vi "BonOMM-SAOMM.Test.vi"() -> ()   [LabVIEW 2011] (continued)
                n3732 = property on="ImgArray" class="IntGraph (strict)"("Cursor.Cursor Position"=w1831) -> ()  [unwired: 2 in, 2 out]
              }
              event "StartServo": Value Change {
                # "Permet l'annulation des\ncommandes de guidage."
                n3733 = event-data() -> ()  [unwired: 1 in, 5 out]
                n3734 = local write "StartServo"(FALSE ("StartServo")) -> ()
                n3735 = local write "GuidingCancel"(FALSE ("GuidingCancel")) -> ()
                n3736 = Less Or Equal?(x="Mode", y=u16 3) -> (x <= y?=w1870:bool)
                n3737 = case shown="True" w1870 {
                  tunnel: "Mode" -> [_ w1876]
                  frame False {
                    # "Ici, ce sera le mode \"calibration\" ..."
                  }
                  frame True {
                    # "Pour lancer le guidage traditionnel, il suffit de\nmettre l'indicateur d'activation à \"vrai\" ... on en\nprofite aussi pour remettre le compteur à zéro."
                    n3738 = flat-sequence {
                      tunnel: w1876 -> [w1879]
                      tunnel: [w1879] -> w1875
                      tunnel: [w1877] -> w1872
                      tunnel: w1875 -> [w1895]
                      tunnel: [w1895] -> w1874
                      tunnel: w1872 -> [w1894]
                      tunnel: w1874 -> [w1906]
                      tunnel: [w1906] -> w1873
                      tunnel: w1873 -> [w1944]
                      frame #0 {
                        w1882 = T17."Disabled and Grayed Out" ("Disabled")
                        w1884 = T17."Disabled" ("Disabled")
                        # "Si le mode est calibration\nC'est qu'on ajuste la collimation"
                        # "Lors de offset, un fichier sera créer à chaque fois :("
                        n3739 = local read "LoggingTimeStamp"() -> (→"GraphTimeStamp":dbl)
                        n3740 = Get Date/Time In Seconds() -> (seconds since 1Jan1904=w1888:timestamp)
                        n3741 = To Double Precision Float(number=w1888) -> (double precision float=w1889:dbl)
                        n3742 = call "GetPathFromTimeStamp.vi"("UTC Time"=TRUE, "LocalTimeStamp"=w1889, "Changement de date à midi ?"=TRUE) -> ("Time String"=w1886:string)  [unwired: 11 in, 1 out]
                        n3743 = Concatenate Strings(w1886, ".gud") -> (→"TrackLogFilename":string)
                        n3744 = property on="StopCam" class="Bool (strict)"("DisabledEnum"=w1882) -> ()  [unwired: 2 in, 2 out]
                        n3745 = property on="StartServo" class="Bool (strict)"("DisabledEnum"=w1882) -> ()  [unwired: 2 in, 2 out]
                        n3746 = property on="AutoCentroid" class="Bool (strict)"("DisabledEnum"=w1882) -> ()  [unwired: 2 in, 2 out]
                        n3747 = local write "Flux Min"(inf ("Flux Min")) -> ()
                        n3748 = local write "Flux Max"(0.0 ("Flux Max")) -> ()
                        n3749 = property on="Mode" class="Ring (strict)"("DisabledEnum"=w1884) -> ()  [unwired: 2 in, 2 out]
                        n3750 = property on="XReference" class="DigNum (strict)"("DisabledEnum"=w1884) -> ()  [unwired: 2 in, 2 out]
                        n3751 = Equal?(x=u16 3, y=w1879) -> (x = y?=w1880:bool)
                        n3752 = property on="Milieu" class="Bool (strict)"("DisabledEnum"=w1882) -> ()  [unwired: 2 in, 2 out]
                        n3753 = property on="GoCam" class="Bool (strict)"("DisabledEnum"=w1882) -> ()  [unwired: 2 in, 2 out]
                        n3754 = property on="GetOptimal" class="Bool (strict)"("DisabledEnum"=w1882) -> ()  [unwired: 2 in, 2 out]
                        n3755 = property on="YReference" class="DigNum (strict)"("DisabledEnum"=w1884) -> ()  [unwired: 2 in, 2 out]
                        n3756 = property on="exptime" class="DigNum (strict)"("DisabledEnum"=w1884) -> ()  [unwired: 2 in, 2 out]
                        n3757 = Select(t=u16 1, s=w1880, f=w1879) -> (s? t:f=w1877:u16)
                      }
                      frame #1 {
                        n3758 = control-ref of="PrAMS-ACK"() -> (w1900:refnum<vi>)
                        n3759 = control-ref of="PrAMS actif"() -> (w1901:refnum<vi>)
                        n3760 = local read "PrAMS VRN"() -> (w1903:refnum<visa-resource-name>)
                        n3761 = local read "PrAMS Error"() -> (w1902:errorcluster)
                        n3762 = local read "MessageType"() -> (w1899:cluster{string[], u32[]})
                        n3763 = local read "Signature"() -> (w1896:u32)
                        n3764 = call-poly "SAOMM-Num2littleEndian.vi"("Number"=w1894) -> ("LiitleEndianedData"=w1897:u8[])  [unwired: 14 in]
                        n3765 = call "SAOMM-SendSET.vi"("PRAMMS-COMM IN"=w1903, "Active Refnum"=w1901, "PrAMS-ACK"=w1900, "Signature"=w1896, "Error IN"=w1902, "MessageType"=w1899, "Active SET"="emtSetTelescopeServoLevel", "Value (little endianed byte array)"=w1897) -> ("PRAMMS-COMM OUT"=w1905:refnum<visa-resource-name>, "Error OUT"=w1904:errorcluster)  [unwired: 4 in, 2 out]
                        n3766 = local write "PrAMS Error"(w1904) -> ()
                        n3767 = local write "PrAMS VRN"(w1905) -> ()
                      }
                      frame #2 {
                        n3768 = case shown="1" w1906 {
                          frame Default {
                          }
                          frame 0 {
                            w1907 = 1.0
                            n3769 = control-ref of="TCS actif"() -> (w1913:refnum<vi>)
                            n3770 = local read "TCS VRN"() -> (w1910:refnum<visa-resource-name>)
                            n3771 = Build Array(w1907) -> (w1911:dbl[])
                            n3772 = expression code="1000/x"(w1907) -> (w1908:dbl)
                            n3773 = call "EXCOM-CMD.vi"("VRN IN"=w1910, "Bool Refnum"=w1913, "Commande #"=15, "Args"=w1911) -> ("VRN OUT"=w1909:refnum<visa-resource-name>)  [unwired: 9 in, 2 out]
                            n3774 = local write "CorrID"(u64 0 ("CorrID")) -> ()
                            n3775 = local write "Servo"(TRUE ("Servo")) -> ()
                            n3776 = local write "TCS VRN"(w1909) -> ()
                            n3777 = local write "RateDEC"(w1908) -> ()
                            n3778 = local write "RateRA"(w1908) -> ()
                          }
                          frame 1 {
                            w1917 = 1.0
                            # "Dans le cas 1, on fonctionne aussi en guidage\ntraditionnel avec un GuiderRate de 1\"/s"
                            n3779 = control-ref of="TCS actif"() -> (w1923:refnum<vi>)
                            n3780 = local read "TCS VRN"() -> (w1920:refnum<visa-resource-name>)
                            n3781 = Build Array(w1917) -> (w1921:dbl[])
                            n3782 = expression code="1000/x"(w1917) -> (w1918:dbl)
                            n3783 = call "EXCOM-CMD.vi"("VRN IN"=w1920, "Bool Refnum"=w1923, "Commande #"=15, "Args"=w1921) -> ("VRN OUT"=w1919:refnum<visa-resource-name>)  [unwired: 9 in, 2 out]
                            n3784 = local write "CorrID"(u64 0 ("CorrID")) -> ()
                            n3785 = local write "TCS VRN"(w1919) -> ()
                            n3786 = local write "RateDEC"(w1918) -> ()
                            n3787 = local write "RateRA"(w1918) -> ()
                          }
                          frame 2 {
                            # "Dans le cas \"2\", on doit modifier la vitesse de guidage\npour l'ajuster au temps d'exposition de la falcon ..."
                            n3788 = local read "exptime"() -> (w1936:dbl)
                            n3789 = Greater?(x=w1936, y=1.25) -> (0:w1934:bool)
                            n3790 = case shown="True" w1934 {
                              frame False {
                              }
                              frame True {
                                n3791 = One Button Dialog(message="Il est fortement conseillé de ne pas utiliser un temps de pose\nde plus de 1.25 secondes pour l'asservissement actif.\n\nAu delà de 3 secondes, le système se comportera très mal.\n\nAssurez-vous que c'est bien ce que vous voulez faire, dans\nle cas contraire, utiliser plutôt le guidage traditionnel." ("Active SET"), button name ("OK")="J'ai lu le message, merci.") -> ()  [unwired: 1 out]
                              }
                            }
                            n3792 = formula code="GuideRate = 0.1288/(2*exptime);\nMillisecondRate=1000/GuideRate;"("exptime"=w1936) -> ("GuideRate"=w1927:dbl, "MillisecondRate"=w1924:dbl)
                            n3793 = In Range and Coerce(upper limit=1.0, x=w1927, lower limit=0.05) -> (coerced(x)=w1928:dbl)  [unwired: 1 out]
                            n3794 = control-ref of="TCS actif"() -> (w1933:refnum<vi>)
                            n3795 = local read "TCS VRN"() -> (w1930:refnum<visa-resource-name>)
                            n3796 = Build Array(w1928) -> (w1931:dbl[])
                            n3797 = call "EXCOM-CMD.vi"("VRN IN"=w1930, "Bool Refnum"=w1933, "Commande #"=15, "Args"=w1931) -> ("VRN OUT"=w1929:refnum<visa-resource-name>)  [unwired: 9 in, 2 out]
                            n3798 = local write "RateDEC"(w1924) -> ()
                            n3799 = local write "TCS VRN"(w1929) -> ()
                            n3800 = local write "RateRA"(w1924) -> ()
                          }
                          frame 3 {
                            n3801 = local write "CorrID"(u64 18446744073709551615 ("CorrID")) -> ()
                          }
                        }
                      }
                      frame #3 {
                        n3802 = local read "XReference"() -> (w1962:dbl)
                        n3803 = local read "YReference"() -> (w1956:dbl)
                        n3804 = local read "Position X"() -> (w1946:dbl)
                        n3805 = local read "Position Y"() -> (w1945:dbl)
                        n3806 = Number To Decimal String(number=w1944) -> (decimal integer string=w1941:string)  [unwired: 1 in]
                        n3807 = Number To Fractional String(number=w1962, precision (6)=i16 1) -> (F-format string=w1963:string)  [unwired: 2 in]
                        n3808 = Number To Fractional String(number=w1956, precision (6)=i16 1) -> (F-format string=w1958:string)  [unwired: 2 in]
                        n3809 = Number To Fractional String(number=w1946, precision (6)=i16 0) -> (F-format string=w1950:string)  [unwired: 2 in]
                        n3810 = Number To Fractional String(number=w1945, precision (6)=i16 0) -> (F-format string=w1954:string)  [unwired: 2 in]
                        n3811 = Concatenate Strings("Pixels de référence [X, Y] : [", w1963, ", ", w1958, "]") -> (w1948:string)
                        n3812 = Concatenate Strings("Position des tables [X, Y, Z] : ", w1950, ", ", w1954, "]") -> (w1947:string)
                        n3813 = Concatenate Strings("Lancement de l'asservissement (mode = '", w1941, "')") -> (w1940:string)
                        n3814 = Build Array(w1940, w1948, w1947) -> (w1965:string[])
                        n3815 = for {
                          tunnel: w1965 -> [w1966] mode=indexing
                          n3816 = control-ref of="TERMINAL"() -> (w1968:refnum<vi>)
                          n3817 = control-ref of="Indicateur d'état"() -> (w1967:refnum<vi>)
                          n3818 = call "TERMINAL.vi"("Indicateur Refnum"=w1967, "Terminal Refnum"=w1968, "Indicateur d'état"=w1966) -> ()
                        }
                      }
                    }
                  }
                }
              }
              event "StopServo": Value Change {
                n3819 = event-data() -> ()  [unwired: 1 in, 5 out]
                n3820 = local write "StopServo"(FALSE ("StopServo")) -> ()
                n3821 = flat-sequence {
                  frame #0 {
                    # "Quand le mode '0' est actif,\nPrAMS n'est pas au courant\net n'enverra l'événement \n\"emtTelescopeServoLevelChanged\""
                    n3822 = local read "Mode"() -> (w1970:u16)
                    n3823 = case shown="0" w1970 {
                      frame Default {
                      }
                      frame 0 {
                        n3824 = local write "Servo"(FALSE ("StopServo")) -> ()
                      }
                    }
                  }
                  frame #1 {
                    w1972 = u16 0 items=["Opération Fixe", "Asservissement Ouvert", "Asservissement Fermé", "Calibration"] ("Mode")
                    n3825 = local read "PrAMS VRN"() -> (w1980:refnum<visa-resource-name>)
                    n3826 = local read "PrAMS Error"() -> (w1979:errorcluster)
                    n3827 = local read "MessageType"() -> (w1976:cluster{string[], u32[]})
                    n3828 = control-ref of="PrAMS-ACK"() -> (w1977:refnum<vi>)
                    n3829 = control-ref of="PrAMS actif"() -> (w1978:refnum<vi>)
                    n3830 = local read "Signature"() -> (w1973:u32)
                    n3831 = call-poly "SAOMM-Num2littleEndian.vi"("Number"=w1972) -> ("LiitleEndianedData"=w1974:u8[])  [unwired: 14 in]
                    n3832 = call "SAOMM-SendSET.vi"("PRAMMS-COMM IN"=w1980, "Active Refnum"=w1978, "PrAMS-ACK"=w1977, "Signature"=w1973, "Error IN"=w1979, "MessageType"=w1976, "Active SET"="emtSetTelescopeServoLevel", "Value (little endianed byte array)"=w1974) -> ("PRAMMS-COMM OUT"=w1982:refnum<visa-resource-name>, "Error OUT"=w1981:errorcluster)  [unwired: 4 in, 2 out]
                    n3833 = local write "PrAMS Error"(w1981) -> ()
                    n3834 = local write "PrAMS VRN"(w1982) -> ()
                  }
                  frame #2 {
                    w1983 = TRUE
                    w1984 = T17."Enabled" ("Disabled")
                    n3835 = property on="StopCam" class="Bool (strict)"("DisabledEnum"=w1984) -> ()  [unwired: 2 in, 2 out]
                    n3836 = property on="StartServo" class="Bool (strict)"("DisabledEnum"=w1984) -> ()  [unwired: 2 in, 2 out]
                    n3837 = property on="XReference" class="DigNum (strict)"("DisabledEnum"=w1984) -> ()  [unwired: 2 in, 2 out]
                    n3838 = local write "ForceSaveToFile"(w1983) -> ()
                    n3839 = local write "GuidingCancel"(w1983) -> ()
                    n3840 = property on="GoCam" class="Bool (strict)"("DisabledEnum"=w1984) -> ()  [unwired: 2 in, 2 out]
                    n3841 = property on="YReference" class="DigNum (strict)"("DisabledEnum"=w1984) -> ()  [unwired: 2 in, 2 out]
                    n3842 = property on="Mode" class="Ring (strict)"("DisabledEnum"=w1984) -> ()  [unwired: 2 in, 2 out]
                    n3843 = property on="Milieu" class="Bool (strict)"("DisabledEnum"=w1984) -> ()  [unwired: 2 in, 2 out]
                    n3844 = property on="exptime" class="DigNum (strict)"("DisabledEnum"=w1984) -> ()  [unwired: 2 in, 2 out]
                    n3845 = property on="AutoCentroid" class="Bool (strict)"("DisabledEnum"=w1984) -> ()  [unwired: 2 in, 2 out]
                    n3846 = property on="GetOptimal" class="Bool (strict)"("DisabledEnum"=w1984) -> ()  [unwired: 2 in, 2 out]
                  }
                  frame #3 {
                    w1985 = inf
                    n3847 = Initialize Array(0.0, 0) -> (w1995:dbl[])
                    n3848 = control-ref of="TCS actif"() -> (w1990:refnum<vi>)
                    n3849 = local read "TCS VRN"() -> (w1987:refnum<visa-resource-name>)
                    n3850 = Bundle(w1995, w1995) -> (w1993:cluster{dbl[], dbl[]})  [unwired: 1 in]
                    n3851 = Build Array(1.0 ("element")) -> (w1988:dbl[])
                    n3852 = Initialize Array(w1993, 0) -> (w1992:cluster{dbl[], dbl[]}[])
                    n3853 = local write "DiffX"(w1985) -> ()
                    n3854 = call "EXCOM-CMD.vi"("VRN IN"=w1987, "Bool Refnum"=w1990, "Commande #"=15, "Args"=w1988) -> ("VRN OUT"=w1986:refnum<visa-resource-name>)  [unwired: 9 in, 2 out]
                    n3855 = local write "Graph-Flux"(w1992) -> ()
                    n3856 = local write "Graph-Centroids"(w1992) -> ()
                    n3857 = local write "Graph-SNR"(w1992) -> ()
                    n3858 = local write "TCS VRN"(w1986) -> ()
                    n3859 = local write "DiffY"(w1985) -> ()
                    n3860 = local write "Hex-XGraph"(w1992) -> ()
                    n3861 = local write "Hex-YGraph"(w1992) -> ()
                    n3862 = local write "Guiderreur"(w1992) -> ()
                    n3863 = local write "Cumulatif"(w1992) -> ()
                  }
                }
              }
              event "SendHexOffset": Value Change {
                n3864 = event-data() -> ()  [unwired: 1 in, 5 out]
                n3865 = local write "SendHexOffset"(FALSE ("SendHexOffset")) -> ()
                n3866 = local read "MessageType"() -> (w2023:cluster{string[], u32[]})
                n3867 = local read "Hexapod VRN"() -> (w2030:refnum<visa-resource-name>)
                n3868 = control-ref of="HexaCons actif"() -> (w2031:refnum<vi>)
                n3869 = control-ref of="Hexapod-ACK"() -> (w2029:refnum<vi>)
                n3870 = local read "PrAMS Error"() -> (w2032:errorcluster)
                n3871 = call-poly "SAOMM-Num2littleEndian.vi"("Number"="Offset X") -> ("LiitleEndianedData"=w2015:u8[])  [unwired: 14 in]
                n3872 = call-poly "SAOMM-Num2littleEndian.vi"("Number"="Offset Y") -> ("LiitleEndianedData"=w2010:u8[])  [unwired: 14 in]
                n3873 = call-poly "SAOMM-Num2littleEndian.vi"("Number"="Offset Z") -> ("LiitleEndianedData"=w2009:u8[])  [unwired: 14 in]
                n3874 = call-poly "SAOMM-Num2littleEndian.vi"("Number"="Offset U") -> ("LiitleEndianedData"=w2006:u8[])  [unwired: 14 in]
                n3875 = call-poly "SAOMM-Num2littleEndian.vi"("Number"="Offset V") -> ("LiitleEndianedData"=w2005:u8[])  [unwired: 14 in]
                n3876 = local read "Signature"() -> (w2026:u32)
                n3877 = call "SAOMM-SendSET.vi"("PRAMMS-COMM IN"=w2030, "Active Refnum"=w2031, "PrAMS-ACK"=w2029, "Signature"=w2026, "Error IN"=w2032, "MessageType"=w2023, "Active SET"="emtSetXAxisOffset", "Value (little endianed byte array)"=w2015) -> ("PRAMMS-COMM OUT"=w2028:refnum<visa-resource-name>, "Error OUT"=w2019:errorcluster)  [unwired: 4 in, 2 out]
                n3878 = call "SAOMM-SendSET.vi"("PRAMMS-COMM IN"=w2028, "Active Refnum"=w2031, "PrAMS-ACK"=w2029, "Signature"=w2026, "Error IN"=w2019, "MessageType"=w2023, "Active SET"="emtSetYAxisOffset", "Value (little endianed byte array)"=w2010) -> ("PRAMMS-COMM OUT"=w2027:refnum<visa-resource-name>, "Error OUT"=w2020:errorcluster)  [unwired: 4 in, 2 out]
                n3879 = call "SAOMM-SendSET.vi"("PRAMMS-COMM IN"=w2027, "Active Refnum"=w2031, "PrAMS-ACK"=w2029, "Signature"=w2026, "Error IN"=w2020, "MessageType"=w2023, "Active SET"="emtSetZAxisOffset", "Value (little endianed byte array)"=w2009) -> ("PRAMMS-COMM OUT"=w1999:refnum<visa-resource-name>, "Error OUT"=w2021:errorcluster)  [unwired: 4 in, 2 out]
                n3880 = call "SAOMM-SendSET.vi"("PRAMMS-COMM IN"=w1999, "Active Refnum"=w2031, "PrAMS-ACK"=w2029, "Signature"=w2026, "Error IN"=w2021, "MessageType"=w2023, "Active SET"="emtSetUAxisOffset", "Value (little endianed byte array)"=w2006) -> ("PRAMMS-COMM OUT"=w1998:refnum<visa-resource-name>, "Error OUT"=w2022:errorcluster)  [unwired: 4 in, 2 out]
                n3881 = call "SAOMM-SendSET.vi"("PRAMMS-COMM IN"=w1998, "Active Refnum"=w2031, "PrAMS-ACK"=w2029, "Signature"=w2026, "Error IN"=w2022, "MessageType"=w2023, "Active SET"="emtSetVAxisOffset", "Value (little endianed byte array)"=w2005) -> ("PRAMMS-COMM OUT"=w2000:refnum<visa-resource-name>, "Error OUT"=w2001:errorcluster)  [unwired: 4 in, 2 out]
                n3882 = case shown="No Error" w2001 {
                  selector: w2001 -> [w2035 w2044]
                  tunnel: w2031 -> [w2043 _]
                  tunnel: w2029 -> [w2042 _]
                  tunnel: w2026 -> [w2041 _]
                  tunnel: [w2040 w2045] -> w2025
                  tunnel: [w2039 w2044] -> w2024
                  tunnel: w2023 -> [w2038 _]
                  tunnel: "emtApplyAxesOffsets" -> [w2037 _]
                  tunnel: u8[] [] ("Value (little endianed byte array)") -> [w2036 _]
                  tunnel: w2000 -> [w2034 w2045]
                  frame No Error {
                    n3883 = call "SAOMM-SendSET.vi"("PRAMMS-COMM IN"=w2034, "Active Refnum"=w2043, "PrAMS-ACK"=w2042, "Signature"=w2041, "Error IN"=w2035, "MessageType"=w2038, "Active SET"=w2037, "Value (little endianed byte array)"=w2036) -> ("PRAMMS-COMM OUT"=w2040:refnum<visa-resource-name>, "Error OUT"=w2039:errorcluster)  [unwired: 4 in, 2 out]
                  }
                  frame Error {
                  }
                }
                n3884 = local write "Hexapod VRN"(w2025) -> ()
                n3885 = local write "PrAMS Error"(w2024) -> ()
              }
              event "HexRAZ": Value Change {
                n3886 = event-data() -> ()  [unwired: 1 in, 5 out]
                n3887 = local read "Signature"() -> (w2053:u32)
                n3888 = control-ref of="Hexapod-ACK"() -> (w2055:refnum<vi>)
                n3889 = local read "Hexapod VRN"() -> (w2054:refnum<visa-resource-name>)
                n3890 = local read "PrAMS Error"() -> (w2052:errorcluster)
                n3891 = local read "MessageType"() -> (w2051:cluster{string[], u32[]})
                n3892 = control-ref of="HexaCons actif"() -> (w2056:refnum<vi>)
                n3893 = local read "HexU"() -> (w2050:dbl)
                n3894 = local read "HexV"() -> (w2049:dbl)
                n3895 = local write "HexRAZ"(FALSE ("HexRAZ")) -> ()
                n3896 = call "SAOMM-RaZ.vi"("PRAMMS-COMM IN"=w2054, "Active Refnum"=w2056, "PrAMS-ACK"=w2055, "Signature"=w2053, "Error IN"=w2052, "MessageType"=w2051, "Position U"=w2050, "Position V"=w2049) -> ("PRAMMS-COMM OUT"=w2048:refnum<visa-resource-name>, "Error OUT"=w2047:errorcluster)  [unwired: 6 in]
                n3897 = local write "Hexapod VRN"(w2048) -> ()
                n3898 = local write "PrAMS Error"(w2047) -> ()
              }
            }
            n3899 = local read "Quit"() -> (w1369:bool)
          }
          "PrAMS + SAOMM" <- w949
          n3900 = while {
            shift-right: [w2068] -> _
            shift-left: w959 -> [w2067]
            tunnel: w958 -> [w2063]
            tunnel: [w2061] -> w948
            i -> [w2057]
            stop <- w2061 stop-if-true
            # "ms to wait for 1st 4 bytes"
            n3901 = local read "MessageType"() -> (w2070:cluster{string[], u32[]})
            n3902 = local read "Signature"() -> (w2062:u32)
            n3903 = local read "PrAMS VRN"() -> (w2073:refnum<visa-resource-name>)
            n3904 = local read "PrAMS Error"() -> (w2072:errorcluster)
            n3905 = call "PRAMMS-LISTENER.vi"("PRAMMS-COMM IN"=w2073, "Bool Refnum"=w2063, "MessageTypeArray"=w2070, "Signature"=w2062, "Error IN"=w2072, "ReadTimeOut"=4) -> ("Type"=w2065:string, "ByteArray"=w2069:u8[], "Received?"=w2071:bool)  [unwired: 4 in, 3 out]
            n3906 = flat-sequence {
              tunnel: w2071 -> [w2077]
              tunnel: w2069 -> [w2076]
              tunnel: w2065 -> [w2075]
              tunnel: w2057 -> [w2074]
              frame #0 {
                # "Lit toujours le socket prams et rafraichi l'image s'il s'agît d'une image ..."
                n3907 = case shown="True" w2077 {
                  tunnel: w2075 -> [_ w2080]
                  tunnel: w2076 -> [_ w2079]
                  tunnel: w2074 -> [_ w2078]
                  frame False {
                  }
                  frame True {
                    n3908 = case shown="\"emtFalconImage\"" w2080 {
                      selector: w2080 -> [w2082 _ _ _ _ _ _ _ _ _ _ _ _ _ _ _ _ _ _ _ _ _ _ w2371 _]
                      tunnel: w2079 -> [w2081 w2094 _ _ _ w2119 w2127 w2154 w2173 w2177 w2181 w2202 w2222 w2227 w2234 w2239 w2246 w2253 _ _ w2267 w2273 w2332 w2368 w2392]
                      tunnel: w2078 -> [_ _ _ _ _ _ _ _ _ _ _ _ _ _ _ _ _ _ _ _ _ _ _ _ w2380]
                      frame "Unknown", Default {
                        w2085 = "\r"
                        n3909 = Type Cast(type=w2085, x=w2081) -> (*(type *) &x=w2084:string)
                        n3910 = local read "Dump"() -> (w2087:string)
                        n3911 = Concatenate Strings(w2087, w2082, " : " ("string"), w2084, w2085) -> (→"Dump":string)
                      }
                      frame "emtError" {
                        # "Tableau d'exception qui ne causeront\npas l'affichage d'un message d'erreur."
                        n3912 = To Unsigned Long Integer(number=u32 0) -> (unsigned 32bit integer=w2096:u32)
                        n3913 = call-poly "SAOMM-EXTRACT-DATA.vi"("UINT32"=w2096, "Data"=w2094) -> ("Value"=w2091:u32)  [unwired: 10 in, 3 out]
                        n3914 = Search 1D Array(1D array=u32[] [64], element=w2091) -> (index of element=w2088:i32)  [unwired: 1 in]
                        n3915 = Less Than 0?(x=w2088) -> (x < 0?=w2089:bool)
                        n3916 = case shown="True" w2089 {
                          tunnel: w2091 -> [_ w2100]
                          frame False {
                          }
                          frame True {
                            n3917 = Not Equal To 0?(x=w2100) -> (x != 0?=w2104:bool)
                            n3918 = case shown="False" w2104 {
                              tunnel: w2100 -> [_ w2111]
                              tunnel: ["Erreur reçu de PrAMS (code : indéfini)" w2107] -> w2105
                              frame False {
                              }
                              frame True {
                                n3919 = Number To Decimal String(number=w2111) -> (decimal integer string=w2110:string)  [unwired: 1 in]
                                n3920 = Concatenate Strings("Erreur reçu de PrAMS (code : ", w2110, ")") -> (w2107:string)
                              }
                            }
                            n3921 = local read "FIFO d'erreur"() -> (w2101:T7)
                            n3922 = call "Error_Format.vi"("FIFO IN"=w2101, "Error Code IN"=w2100, "Source"="PrAMS", "Comment"=w2105) -> ("FIFO OUT"=w2102:T7)  [unwired: 13 in, 2 out]
                            n3923 = local write "FIFO d'erreur"(w2102) -> ()
                          }
                        }
                        n3924 = To Long Integer(number=w2091) -> (32bit integer=w2092:i32)
                        n3925 = Negate(x=w2092) -> (-x=w2093:i32)
                        n3926 = local write "PrAMS-ACK"(w2093) -> ()
                        n3927 = local read "Nb_Error (PrAMS)"() -> (w2098:i32)
                        n3928 = Increment(x=w2098) -> (x+1=w2097:i32)
                        n3929 = local write "Nb_Error (PrAMS)"(w2097) -> ()
                        "PrAMS-Error" <- TRUE ("PrAMS-Error")
                      }
                      frame "emtAreYouThere" {
                      }
                      frame "emtAcknowledgment" {
                        n3930 = local read "Nb_ACK (PrAMS)"() -> (w2113:i32)
                        n3931 = Increment(x=w2113) -> (x+1=→"Nb_ACK (PrAMS)":i32)
                        "PrAMS-ACK" <- 1 ("PrAMS-ACK")
                      }
                      frame "emtClientType" {
                        # "Jamais reçu par BonOMM actuellement puisque BonOMM n'envoit pas de \"emtGetClientType\"\n\nEn fait, peut-être qu'il manque un \"Set\" dans l'enum ... genre \"emtSetClientType\""
                      }
                      frame "emtImageExposureTime" {
                        n3932 = To Unsigned Long Integer(number=u32 0) -> (unsigned 32bit integer=w2118:u32)
                        n3933 = call-poly "SAOMM-EXTRACT-DATA.vi"("UINT32"=w2118, "Data"=w2119) -> ("Value"=w2117:u32)  [unwired: 10 in, 3 out]
                        n3934 = To Double Precision Float(number=w2117) -> (double precision float=w2116:dbl)
                        n3935 = expression code="x/1000."(w2116) -> (w2115:dbl)
                        n3936 = local write "exptime"(w2115) -> ()
                      }
                      frame "emtOptimalExposureTime" {
                        n3937 = flat-sequence {
                          tunnel: w2127 -> [w2133]
                          tunnel: [w2130] -> w2125
                          tunnel: [w2129] -> w2123
                          tunnel: [w2128] -> w2121
                          tunnel: [w2140] -> w2126
                          tunnel: w2125 -> [w2140]
                          tunnel: [w2139] -> w2124
                          tunnel: w2123 -> [w2139]
                          tunnel: [w2138] -> w2122
                          tunnel: w2121 -> [w2138]
                          tunnel: w2126 -> [w2146]
                          tunnel: w2124 -> [w2145]
                          tunnel: w2122 -> [w2144]
                          frame #0 {
                            n3938 = To Unsigned Long Integer(number=u32 0) -> (unsigned 32bit integer=w2136:u32)
                            n3939 = call-poly "SAOMM-EXTRACT-DATA.vi"("UINT32"=w2136, "Data"=w2133) -> ("Value"=w2135:u32)  [unwired: 10 in, 3 out]
                            n3940 = To Double Precision Float(number=w2135) -> (double precision float=w2134:dbl)
                            n3941 = expression code="x/1000."(w2134) -> (w2129:dbl)
                            n3942 = In Range and Coerce(upper limit=30.0, x=w2129, lower limit=0.0) -> (coerced(x)=w2128:dbl, In Range?=w2130:bool)
                          }
                          frame #1 {
                            n3943 = local read "GetOptimalTime"() -> (w2142:u32)
                            n3944 = Tick Count (ms)() -> (millisecond timer value=w2141:u32)
                            n3945 = Subtract(x=w2141, y=w2142) -> (x-y=w2143:u32)
                            n3946 = local write "GetOptimalTime"(w2143) -> ()
                          }
                          frame #2 {
                            n3947 = case shown="True" w2146 {
                              tunnel: w2145 -> [w2147 _]
                              tunnel: w2144 -> [_ w2153]
                              frame False {
                                n3948 = Number To Fractional String(number=w2147, precision (6)=i16 2) -> (F-format string=w2151:string)  [unwired: 2 in]
                                n3949 = Concatenate Strings("La valeur optimale retournée (", w2151, ") est hors de l'intervalle acceptée.") -> (w2148:string)
                                n3950 = One Button Dialog(message=w2148) -> ()  [unwired: 1 in, 1 out]
                              }
                              frame True {
                                # "On envoit la nouvelle valeur comme valeur actuelle"
                                n3951 = property on="exptime" class="DigNum (strict)"("Val(Sgnl)"=w2153) -> ()  [unwired: 2 in, 2 out]
                              }
                            }
                          }
                        }
                      }
                      frame "emtImageEMGain" {
                        n3952 = flat-sequence {
                          tunnel: w2154 -> [w2156]
                          frame #0 {
                            n3953 = To Unsigned Word Integer(number=u16 0) -> (unsigned 16bit integer=w2157:u16)
                            n3954 = call-poly "SAOMM-EXTRACT-DATA.vi"("UINT16"=w2157, "Data"=w2156) -> ("Value"=→"EMGain":u16)  [unwired: 10 in, 3 out]
                          }
                          frame #1 {
                            n3955 = local read "QueryingPraMS"() -> (w2159:bool)
                            n3956 = case shown="True" w2159 {
                              frame False {
                              }
                              frame True {
                                n3957 = local read "FalconQuery"() -> (w2162:u32)
                                n3958 = Tick Count (ms)() -> (millisecond timer value=w2163:u32)
                                n3959 = Subtract(x=w2163, y=w2162) -> (x-y=w2161:u32)
                                n3960 = local write "QueryingPraMS"(FALSE ("Querying")) -> ()
                                n3961 = local write "FalconQuery"(w2161) -> ()
                              }
                            }
                          }
                        }
                      }
                      frame "emtFPGACtrl" {
                        n3962 = To Unsigned Word Integer(number=u16 0) -> (unsigned 16bit integer=w2171:u16)
                        n3963 = call-poly "SAOMM-EXTRACT-DATA.vi"("UINT16"=w2171, "Data"=w2173) -> ("Value"=w2165:u16)  [unwired: 10 in, 3 out]
                        "FPGA Value" <- w2165
                        n3964 = Number To Decimal String(number=w2165) -> (decimal integer string=w2168:string)  [unwired: 1 in]
                        n3965 = control-ref of="TERMINAL"() -> (w2169:refnum<vi>)
                        n3966 = control-ref of="Indicateur d'état"() -> (w2170:refnum<vi>)
                        n3967 = Concatenate Strings("FAPG.get -> (", w2168, ")" ("string")) -> (w2164:string)
                        n3968 = call "TERMINAL.vi"("Indicateur Refnum"=w2170, "Terminal Refnum"=w2169, "Indicateur d'état"=w2164) -> ()
                      }
                      frame "emtImageWidth" {
                        n3969 = To Unsigned Word Integer(number=u16 0) -> (unsigned 16bit integer=w2174:u16)
                        n3970 = call-poly "SAOMM-EXTRACT-DATA.vi"("UINT16"=w2174, "Data"=w2177) -> ("Value"=w2176:u16)  [unwired: 10 in, 3 out]
                        n3971 = local write "ImageWidth"(w2176) -> ()
                      }
                      frame "emtImageHeight" {
                        n3972 = To Unsigned Word Integer(number=u16 0) -> (unsigned 16bit integer=w2178:u16)
                        n3973 = call-poly "SAOMM-EXTRACT-DATA.vi"("UINT16"=w2178, "Data"=w2181) -> ("Value"=w2180:u16)  [unwired: 10 in, 3 out]
                        n3974 = local write "ImageHeight"(w2180) -> ()
                      }
                      frame "emtImageBinning" {
                        w2192 = "cam_Binning "
                        n3975 = To Unsigned Word Integer(number=0) -> (unsigned 16bit integer=w2200:u16)
                        n3976 = call-poly "SAOMM-EXTRACT-DATA.vi"("UINT16"=w2200, "Data"=w2202) -> ("Value"=w2187:u16)  [unwired: 10 in, 3 out]
                        n3977 = local write "Binning"(w2187) -> ()
                        n3978 = case shown="1, Default" w2187 {
                          tunnel: [TRUE FALSE FALSE FALSE] -> w2186
                          tunnel: [FALSE TRUE FALSE FALSE] -> w2185
                          tunnel: [FALSE FALSE TRUE FALSE] -> w2184
                          tunnel: [FALSE FALSE FALSE TRUE] -> w2183
                          frame 1, Default {
                          }
                          frame 2 {
                          }
                          frame 4 {
                          }
                          frame 5 {
                          }
                        }
                        n3979 = Current VI's Menubar() -> (w2182:refnum<k9>)
                        n3980 = Concatenate Strings(w2192, "1x1" ("string")) -> (w2191:string)
                        n3981 = Set Menu Item Info(6:w2186, 7:w2191, 11:w2182) -> (3:w2188:refnum<k9>)  [unwired: 4 in, 1 out]
                        n3982 = Concatenate Strings(w2192, "2x2" ("string")) -> (w2197:string)
                        n3983 = Set Menu Item Info(6:w2185, 7:w2197, 11:w2188) -> (3:w2189:refnum<k9>)  [unwired: 4 in, 1 out]
                        n3984 = Concatenate Strings(w2192, "4x4" ("string")) -> (w2198:string)
                        n3985 = Set Menu Item Info(6:w2184, 7:w2198, 11:w2189) -> (3:w2190:refnum<k9>)  [unwired: 4 in, 1 out]
                        n3986 = Concatenate Strings(w2192, "5x5" ("string")) -> (w2199:string)
                        n3987 = Set Menu Item Info(6:w2183, 7:w2199, 11:w2190) -> ()  [unwired: 4 in, 2 out]
                      }
                      frame "emtImageDisplayFrameRate" {
                        n3988 = To Double Precision Float(number=0.0) -> (double precision float=w2220:dbl)
                        n3989 = call-poly "SAOMM-EXTRACT-DATA.vi"("DBL"=w2220, "Data"=w2222) -> ("Value"=w2219:dbl)  [unwired: 10 in, 3 out]
                        n3990 = local write "ImageFPS"(w2219) -> ()
                      }
                      frame "emtROIWidth" {
                        n3991 = To Unsigned Word Integer(number=u16 0) -> (unsigned 16bit integer=w2225:u16)
                        n3992 = call-poly "SAOMM-EXTRACT-DATA.vi"("UINT16"=w2225, "Data"=w2227) -> ("Value"=w2226:u16, "Min"=→"ROIWidthMin":u16, "Max"=→"ROIWidthMax":u16)  [unwired: 10 in, 1 out]
                        n3993 = local write "ROIWidth"(w2226) -> ()
                      }
                      frame "emtROIHeight" {
                        n3994 = To Unsigned Word Integer(number=u16 0) -> (unsigned 16bit integer=w2231:u16)
                        n3995 = call-poly "SAOMM-EXTRACT-DATA.vi"("UINT16"=w2231, "Data"=w2234) -> ("Value"=w2233:u16, "Min"=→"ROIHeightMin":u16, "Max"=→"ROIHeightMax":u16)  [unwired: 10 in, 1 out]
                        n3996 = local write "ROIHeight"(w2233) -> ()
                      }
                      frame "emtROIXOffset" {
                        n3997 = To Unsigned Word Integer(number=u16 0) -> (unsigned 16bit integer=w2237:u16)
                        n3998 = call-poly "SAOMM-EXTRACT-DATA.vi"("UINT16"=w2237, "Data"=w2239) -> ("Value"=w2238:u16, "Min"=w2236:u16, "Max"=w2235:u16)  [unwired: 10 in, 1 out]
                        n3999 = local write "ROIXOffset"(w2238) -> ()
                        n4000 = local write "ROIXMin"(w2236) -> ()
                        n4001 = local write "ROIXMax"(w2235) -> ()
                      }
                      frame "emtROIYOffset" {
                        n4002 = To Unsigned Word Integer(number=u16 0) -> (unsigned 16bit integer=w2243:u16)
                        n4003 = call-poly "SAOMM-EXTRACT-DATA.vi"("UINT16"=w2243, "Data"=w2246) -> ("Value"=w2244:u16, "Min"=w2242:u16, "Max"=w2241:u16)  [unwired: 10 in, 1 out]
                        n4004 = local write "ROIYOffset"(w2244) -> ()
                        n4005 = local write "ROIYMax"(w2241) -> ()
                        n4006 = local write "ROIYMin"(w2242) -> ()
                      }
                      frame "emtTelescopeServoLevel" {
                        # "En supposant que ça retourne le TelescopeServoLevel"
                        # "Si Level > \"Opération Fixe\"\nAlors c'est que l'asservissement\nest enclenché."
                        # "Reçoit la nouvelle valeur de emtTelescopeServoLevel"
                        n4007 = To Unsigned Long Integer(number=0) -> (unsigned 32bit integer=w2251:u32)
                        n4008 = call-poly "SAOMM-EXTRACT-DATA.vi"("UINT32"=w2251, "Data"=w2253) -> ("Value"=w2250:u32)  [unwired: 10 in, 3 out]
                        n4009 = To Unsigned Word Integer(number=w2250) -> (unsigned 16bit integer=w2249:u16)
                        n4010 = Greater?(x=w2249, y=u16 0) -> (0:w2247:bool)
                        n4011 = local write "Mode"(w2249) -> ()
                        n4012 = local write "Servo"(w2247) -> ()
                        n4013 = case shown="True" w2247 {
                          frame False {
                            # "Réinitialise les variables relatives à l'asservissement\nHistorique, etc ..."
                          }
                          frame True {
                          }
                        }
                      }
                      frame "emtAcquisitionStarted" {
                        w2254 = T17."Enabled" ("Disabled")
                        n4014 = local write "Integrating"(TRUE) -> ()
                        n4015 = property on="Mode" class="Ring (strict)"("DisabledEnum"=w2254) -> ()  [unwired: 2 in, 2 out]
                        n4016 = property on="StartServo" class="Bool (strict)"("DisabledEnum"=w2254) -> ()  [unwired: 2 in, 2 out]
                        n4017 = property on="StopServo" class="Bool (strict)"("DisabledEnum"=w2254) -> ()  [unwired: 2 in, 2 out]
                      }
                      frame "emtAcquisitionStopped" {
                        w2256 = FALSE ("Visible")
                        w2257 = "N/D"
                        w2258 = T17."Disabled and Grayed Out" ("Disabled")
                        w2259 = u16 2 items=["Region d'intérêt", "Prévisualisation", "Idle"] ("ImageUsage")
                        n4018 = property on="Mode" class="Ring (strict)"("DisabledEnum"=w2258) -> ()  [unwired: 2 in, 2 out]
                        n4019 = property on="StartServo" class="Bool (strict)"("DisabledEnum"=w2258) -> ()  [unwired: 2 in, 2 out]
                        n4020 = property on="StopServo" class="Bool (strict)"("DisabledEnum"=w2258) -> ()  [unwired: 2 in, 2 out]
                        n4021 = local write "ImageUsage"(w2259) -> ()
                        n4022 = local write "subimg"(sgl[][] [] ("ImgArray")) -> ()
                        n4023 = local write "Integrating"(FALSE) -> ()
                        n4024 = local write "InstantFPS"(0.0 ("InstantFPS")) -> ()
                        n4025 = property on="LowSNR" class="Bool (strict)"("Visible"=w2256, "Blinking"=w2256) -> ()  [unwired: 2 in, 2 out]
                        n4026 = property on="Saturé" class="Bool (strict)"("Visible"=w2256, "Blinking"=w2256) -> ()  [unwired: 2 in, 2 out]
                        "ImgArray" <- u32[][] [] ("ImgArray")
                        "ErrY" <- w2257
                        "ErrX" <- w2257
                      }
                      frame "emtTelescopeServoLevelChanged" {
                        # "Update la nouvelle valeur pour assurer que c'est le bon."
                        n4027 = local read "Mode"() -> (w2266:u16)
                        n4028 = call-poly "SAOMM-EXTRACT-DATA.vi"("UINT16"=w2266, "Data"=w2267) -> ("Value"=w2264:u16)  [unwired: 10 in, 3 out]
                        n4029 = local write "Mode"(w2264) -> ()
                        n4030 = Greater Than 0?(x=w2264) -> (x > 0?=→"Servo":bool)
                      }
                      frame "emtFalconImage" {
                        n4031 = flat-sequence {
                          tunnel: w2273 -> [w2278]
                          tunnel: [w2278] -> w2272
                          tunnel: [w2277] -> w2270
                          tunnel: [w2275] -> w2269
                          tunnel: [w2274] -> w2268
                          tunnel: w2272 -> [w2300]
                          tunnel: [w2294] -> w2271
                          tunnel: w2270 -> [w2294]
                          tunnel: w2269 -> [w2291]
                          tunnel: w2268 -> [w2290]
                          tunnel: w2271 -> [w2331]
                          frame #0 {
                            n4032 = local read "LastImageID"() -> (w2275:u32)
                            n4033 = local write "Integrating"(TRUE) -> ()
                            n4034 = Get Date/Time In Seconds() -> (seconds since 1Jan1904=w2274:timestamp)
                            n4035 = Tick Count (ms)() -> (millisecond timer value=w2277:u32)
                          }
                          frame #1 {
                            # "Comme il n'y a pas de critères sur le ID, il se peut qu'on recoive la dernière image et non la prochaine ..."
                            n4036 = To Double Precision Float(number=w2290) -> (double precision float=w2283:dbl)
                            n4037 = call "PRAMMS-DataString2Image.vi"("ImageData"=w2300) -> ("Width"=→"ImageWidth":u16, "Height"=→"ImageHeight":u16, "Image"=w2280:u16[][], "ImageID"=w2279:u32)  [unwired: 8 in, 3 out]
                            n4038 = local read "LastImageTime"() -> (w2284:dbl)
                            n4039 = local read "SaveNextImage"() -> (w2282:bool)
                            n4040 = To Unsigned Long Integer(number=w2280) -> (unsigned 32bit integer=w2281:u32[][])
                            n4041 = local write "LastImageID"(w2279) -> ()
                            n4042 = local write "ImgArray"(w2281) -> ()
                            n4043 = local read "TmpFalcon"() -> (w2299:u32)
                            n4044 = case shown="True" w2282 {
                              tunnel: w2280 -> [_ w2323]
                              frame False {
                              }
                              frame True {
                                n4045 = Get Date/Time In Seconds() -> (seconds since 1Jan1904=w2313:timestamp)
                                n4046 = local read "path_data"() -> (w2318:path)
                                n4047 = To Double Precision Float(number=w2313) -> (double precision float=w2312:dbl)
                                n4048 = local write "SaveNextImage"(FALSE ("SaveNextImage")) -> ()
                                n4049 = call "GetPathFromTimeStamp.vi"("UTC Time"=FALSE, "LocalTimeStamp"=w2312, "Changement de date à midi ?"=FALSE) -> ("Date String"=w2317:string, "Time String"=w2316:string)  [unwired: 11 in]
                                n4050 = Concatenate Strings(w2317, w2316, ".fits" ("string")) -> (w2314:string)
                                n4051 = Build Path(base path=w2318, name or relative path=path "CameraImages") -> (appended path=w2320:path)
                                n4052 = local read "Dec Sonde"() -> (w2307:dbl)
                                n4053 = local read "ROIYOffset"() -> (w2304:u16)
                                n4054 = local read "Epoch Tel"() -> (w2306:dbl)
                                n4055 = local read "RA Sonde"() -> (w2308:dbl)
                                n4056 = local read "PixScale2"() -> (w2302:dbl)
                                n4057 = local read "ROIXOffset"() -> (w2303:u16)
                                n4058 = local read "exptime"() -> (w2309:dbl)
                                n4059 = local read "PixScale1"() -> (w2301:dbl)
                                n4060 = local read "Binning"() -> (w2305:u16)
                                n4061 = Build Path(base path=w2320, name or relative path=w2314) -> (appended path=w2321:path)
                                n4062 = call "SaveFalconImage.vi"("SavePath"=w2321, "Binning"=w2305, "ROIYOffset"=w2304, "ROIXOffset"=w2303, "PixScale1"=w2301, "Image"=w2323, "EXPTIME"=w2309, "RA Sonde"=w2308, "Dec Sonde"=w2307, "Epoch Tel"=w2306, "PixScale2"=w2302) -> ()  [unwired: 5 in]
                              }
                            }
                            n4063 = Subtract(x=w2283, y=w2284) -> (x-y=w2287:dbl)
                            n4064 = Greater?(x=w2279, y=w2291) -> (0:w2289:bool)
                            n4065 = Tick Count (ms)() -> (millisecond timer value=w2298:u32)
                            n4066 = flat-sequence {
                              tunnel: w2299 -> [w2328]
                              tunnel: w2298 -> [w2327]
                              tunnel: [w2326] -> w2297
                              frame #0 {
                                n4067 = Subtract(x=w2327, y=w2328) -> (x-y=w2326:u32)
                                "TmpFalcon" <- w2327
                              }
                            }
                            n4068 = Greater?(x=w2287, y=0.5) -> (0:w2285:bool)
                            n4069 = And(x=w2289, y=w2285) -> (x .and. y?=w2288:bool)
                            n4070 = To Double Precision Float(number=w2297) -> (double precision float=w2296:dbl)
                            n4071 = case shown="True" w2288 {
                              selector: w2288 -> [_ w2325]
                              tunnel: w2283 -> [_ w2324]
                              frame False {
                              }
                              frame True {
                                n4072 = property on="FalconProcessed" class="Bool (strict)"("Val(Sgnl)"=w2325) -> ()  [unwired: 2 in, 2 out]
                                "LastImageTime" <- w2324
                              }
                            }
                            n4073 = expression code="1/(x/1000)"(w2296) -> (→"InstantFPS":dbl)
                          }
                          frame #2 {
                            n4074 = Tick Count (ms)() -> (millisecond timer value=w2330:u32)
                            n4075 = Subtract(x=w2330, y=w2331) -> (x-y=→"ImageProcessing":u32)
                          }
                        }
                      }
                      frame "emtProcessedFalconImage" {
                        n4076 = flat-sequence {
                          tunnel: w2332 -> [w2336]
                          frame #0 {
                            w2360 = u16 0 items=["Region d'intérêt", "Prévisualisation"] ("ImageUsage")
                            # "Devrais peut-être servir uniquement à recevoir la sous-image ..."
                            # "Viens pluôt de FalconImage"
                            # "Vérifier le format ..."
                            # "Possiblement ajouter/soustraire 0.5 pixels ..."
                            n4077 = call "SAOMM-ProcImageParser.vi"("ProcessedData"=w2336) -> ("ImageBuffer"=→"ImageBuffer":u16[][], "GrayLevels"=w2334:u8[][], "MaskObjet"=→"MaskObjet":u8[][], "GeneralProperties"=w2345:T52, "ROIProperties"=w2346:T53, "ProcessedProperties"=w2361:T54)  [unwired: 8 in, 1 out]
                            n4078 = Unbundle By Name(w2346) -> ("Position X de la ROI"=w2344:u16)
                            n4079 = Unbundle By Name(w2346) -> ("Position Y de la ROI"=w2342:u16)
                            n4080 = Unbundle By Name(w2361) -> ("Centroide X"=w2343:dbl)
                            n4081 = Unbundle By Name(w2346) -> ("Hauteur de la ROI"=w2358:u16)
                            n4082 = Unbundle By Name(w2361) -> ("Centroide Y"=w2341:dbl)
                            n4083 = Unbundle By Name(w2346) -> ("Largeur de la ROI"=w2359:u16)
                            n4084 = local read "Nb_FalconProc_reçu"() -> (w2339:u32)
                            n4085 = To Single Precision Float(number=w2334) -> (single precision float=w2364:sgl[][])
                            n4086 = Array Max & Min(array=w2364) -> (max value=w2362:sgl)  [unwired: 3 out]
                            n4087 = call "Draw_crosshair.vi"("Image IN"=w2364, "White Value"=w2362) -> ("Image OUT"=w2363:sgl[][])  [unwired: 13 in]
                            n4088 = local write "ROIWidth"(w2359) -> ()
                            n4089 = local write "ROIHeight"(w2358) -> ()
                            n4090 = To Double Precision Float(number=w2344) -> (double precision float=w2352:dbl)
                            n4091 = To Double Precision Float(number=w2342) -> (double precision float=w2351:dbl)
                            n4092 = Increment(x=w2339) -> (x+1=→"Nb_FalconProc_reçu":u32)
                            n4093 = local write "subimg"(w2363) -> ()
                            n4094 = Add(x=w2343, y=w2352) -> (x+y=w2349:dbl)
                            "XCentroid" <- w2349
                            n4095 = Add(x=w2351, y=w2341) -> (x+y=w2350:dbl)
                            "YCentroid" <- w2350
                            n4096 = local read "XReference"() -> (w2348:dbl)
                            n4097 = local write "ROIXOffset"(w2344) -> ()
                            n4098 = local read "YReference"() -> (w2347:dbl)
                            n4099 = local write "ROIYOffset"(w2342) -> ()
                            n4100 = Unbundle By Name(w2345) -> ("ID de l'image"=w2353:u32)
                            n4101 = Subtract(x=w2348, y=w2349) -> (x-y=w2337:dbl)
                            "DiffX" <- w2337
                            n4102 = Subtract(x=w2347, y=w2350) -> (x-y=w2338:dbl)
                            "DiffY" <- w2338
                            n4103 = local write "LastProcID"(w2353) -> ()
                            n4104 = Number To Fractional String(number=w2338, precision (6)=i16 1) -> (F-format string=w2354:string)  [unwired: 2 in]
                            n4105 = Number To Fractional String(number=w2337, precision (6)=i16 1) -> (F-format string=w2355:string)  [unwired: 2 in]
                            n4106 = local write "ErrY"(w2354) -> ()
                            n4107 = local write "ErrX"(w2355) -> ()
                            "ImageUsage" <- w2360
                            "FalconProcData" <- w2336
                          }
                          frame #1 {
                            # "Certaines images entrent après la réception d'un\nacquisition stopped ..."
                            n4108 = local read "Integrating"() -> (w2365:bool)
                            n4109 = case shown="True" w2365 {
                              frame False {
                              }
                              frame True {
                                n4110 = property on="ProcessImage" class="Bool (strict)"("Val(Sgnl)"=TRUE ("Value (Signaling)")) -> ()  [unwired: 2 in, 2 out]
                              }
                            }
                          }
                        }
                      }
                      frame "emtROIXReferencePoint", "emtROIYReferencePoint" {
                        n4111 = To Double Precision Float(number=u16 0) -> (double precision float=w2369:dbl)
                        n4112 = call-poly "SAOMM-EXTRACT-DATA.vi"("DBL"=w2369, "Data"=w2368) -> ("Value"=w2367:dbl)  [unwired: 10 in, 3 out]
                        n4113 = case shown="\"emtROIXReferencePoint\"" w2371 {
                          tunnel: w2367 -> [_ w2373 w2379]
                          frame Default {
                          }
                          frame "emtROIXReferencePoint" {
                            n4114 = local read "ROIXOffset"() -> (w2375:u16)
                            n4115 = To Double Precision Float(number=w2375) -> (double precision float=w2374:dbl)
                            n4116 = Add(x=w2374, y=w2373) -> (x+y=w2372:dbl)
                            n4117 = local write "XReference"(w2372) -> ()
                            "XROIRef" <- w2373
                          }
                          frame "emtROIYReferencePoint" {
                            n4118 = local read "ROIYOffset"() -> (w2378:u16)
                            n4119 = To Double Precision Float(number=w2378) -> (double precision float=w2377:dbl)
                            n4120 = Add(x=w2377, y=w2379) -> (x+y=w2376:dbl)
                            n4121 = local write "YReference"(w2376) -> ()
                            "YROIRef" <- w2379
                          }
                        }
                      }
                      frame "emtHexapodServoCommandLogging" {
                        # "Nombre de secondes entre les\npremiers janvier 1904 et 1970"
                        # "Utilisation des éléments de HexapodServoCommandLogging"
                        n4122 = call "SAOMM-HistoParser.vi"("DataStream"=w2392) -> ("Source cluster"=w2386:T55, "Hexapod cluster"=w2391:T56)  [unwired: 13 in]
                        n4123 = local read "ConsideredLenght"() -> (w2390:i32)
                        n4124 = Unbundle By Name(w2386) -> ("Logging TimeStapmp"=w2384:u64)
                        n4125 = To Double Precision Float(number=w2384) -> (double precision float=w2385:dbl)
                        n4126 = Unbundle By Name(w2386) -> ("SNR"=w2388:dbl)
                        n4127 = expression code="x/1000"(w2385) -> (w2383:dbl)
                        n4128 = To Double Precision Float(number=w2390) -> (double precision float=w2389:dbl)
                        n4129 = Add(x=w2383, y=2082844799.0) -> (x+y=w2381:dbl)
                        n4130 = local write "LoggingTimeStamp"(w2381) -> ()
                        n4131 = Not Equal To 0?(x=w2388) -> (x != 0?=w2387:bool)
                        n4132 = case shown="True" w2387 {
                          tunnel: w2391 -> [_ w2397]
                          tunnel: w2389 -> [_ w2396]
                          tunnel: w2386 -> [_ w2395]
                          tunnel: w2381 -> [_ w2394]
                          tunnel: w2380 -> [_ w2393]
                          frame False {
                          }
                          frame True {
                            n4133 = stacked-sequence {
                              tunnel: w2397 -> [w2457 _ _ w2552]
                              tunnel: w2395 -> [w2462 _ w2491 _]
                              tunnel: w2396 -> [_ _ w2490 w2551]
                              tunnel: [w2426 _ _ _] -> _
                              tunnel: w2394 -> [_ _ w2475 w2545]
                              tunnel: w2393 -> [_ _ _ _]
                              frame #0 {
                                # "Update des valeurs associées à la trame ..."
                                n4134 = Unbundle By Name(w2457) -> ("Hexapod_Nominal"=w2456:dbl[], "Hexapod_Offset"=w2445:dbl[], "Hexapod_LUT"=w2444:dbl[], "Hexapod_ServoX"=w2442:dbl[], "Hexapode_ServoY"=w2441:dbl[], "Hexapod_Console"=→"H_Console":dbl[], "Hexapod_Position"=w2431:dbl[], "Hexapod_Command"=w2437:dbl[])  [unwired: 1 out]
                                "H_Offset" <- w2445
                                "H_LUT" <- w2444
                                "H_Position" <- w2431
                                "H_Command" <- w2437
                                n4135 = Unbundle By Name(w2462) -> ("ServoLevel"=w2426:u16, "ROIXOffset"=w2461:u16, "ROIYOffset"=w2459:u16, "Pixel X"=w2428:dbl, "Pixel Y"=w2430:dbl, "Flux"=w2402:dbl, "SNR"=w2401:dbl, "CentroidX"=w2460:dbl, "CentroidY"=w2458:dbl, "SNRTreshold"=w2400:dbl)
                                "Flux inst." <- w2402
                                n4136 = Greater Or Equal?(x=w2401, y=w2400) -> (x >= y?=w2399:bool)
                                n4137 = Not(x=w2399) -> (.not. x?=w2398:bool)
                                n4138 = Index Array(array=w2441) -> (element=w2439:dbl)  [unwired: 1 in]
                                n4139 = Index Array(array=w2442) -> (element=w2440:dbl)  [unwired: 1 in]
                                n4140 = local write "SNR"(w2401) -> ()
                                n4141 = Build Array(w2440, w2439) -> (→"H_Servo":dbl[])
                                n4142 = property on="LowSNR" class="Bool (strict)"("Visible"=w2398, "Blinking"=w2398) -> ()  [unwired: 2 in, 2 out]
                                n4143 = Index Array(array=w2456) -> (element #1=→"Nominal X":dbl, element #2=→"Nominal Y":dbl, element #3=→"Nominal Z":dbl, element #4=→"Nominal U":dbl, element #5=→"Nominal V":dbl, element #6=→"Nominal W":dbl)  [unwired: 6 in]
                                n4144 = local write "ROIYOffset"(w2459) -> ()
                                n4145 = Index Array(array=w2444) -> (element #1=→"LUT X":dbl, element #2=→"LUT Y":dbl, element #3=→"LUT Z":dbl, element #4=→"LUT U":dbl, element #5=→"LUT V":dbl, element #6=→"LUT W":dbl)  [unwired: 6 in]
                                n4146 = local write "YROIRef"(w2430) -> ()
                                n4147 = local write "ROIXOffset"(w2461) -> ()
                                n4148 = local write "XROIRef"(w2428) -> ()
                                n4149 = local read "Flux Max"() -> (w2405:dbl)
                                n4150 = local read "Flux Min"() -> (w2404:dbl)
                                n4151 = Index Array(array=w2445) -> (element #1=w2455:dbl, element #2=w2454:dbl, element #3=w2453:dbl, element #4=w2452:dbl, element #5=w2451:dbl)  [unwired: 5 in]
                                n4152 = Greater?(x=w2402, y=w2405) -> (0:w2406:bool)
                                n4153 = Less?(x=w2402, y=w2404) -> (x < y?=w2403:bool)
                                n4154 = Index Array(array=w2431) -> (element #1=→"HexX":dbl, element #2=→"HexY":dbl, element #3=→"HexZ":dbl, element #4=→"HexU":dbl, element #5=→"HexV":dbl, element #6=→"HexW":dbl)  [unwired: 6 in]
                                n4155 = local write "Offset X"(w2455) -> ()
